vi "PicoScope4000SetupStreaming.vi"(0 "handle in":i16, 2 "enabled array":i16[](array[numeric]), 3 "Acquisition Settings":T2 {"Time Units" items=["Nanoseconds (ns)", "Microseconds (us)", "Milliseconds (ms)", "Seconds (s)"]; "Down-Sample Mode" items=["None", "Aggregate", "Decimate", "Average"]}, 4 "Buffer and Transfer Settings":T1 {"Down-Sample Mode" items=["None", "Aggregate", "Average"]; "Down Sample Ratio" step=1; "Samples" format="%_6p"}, 5 "error in":errorcluster, 10 "Pointers In":u64[][](array[numeric])) -> (11 "Pointer array":u64[][](array[numeric]), 14 "handle out":i16, 16 "Sample Interval":u32, 17 "sampleIntervalTimeUnits":u32, 19 "error out":errorcluster)   [LabVIEW 2009]
doc: "Set up the data buffers and calls RunStreaming to start the device streaming.\nData will be copied from the driver buffers into the corresponding application buffers using the wrapper dll."
uses:
  ps4000.dll
  ps4000Wrap.dll
  PicoScope4000Buffer and Transfer Settings.ctl
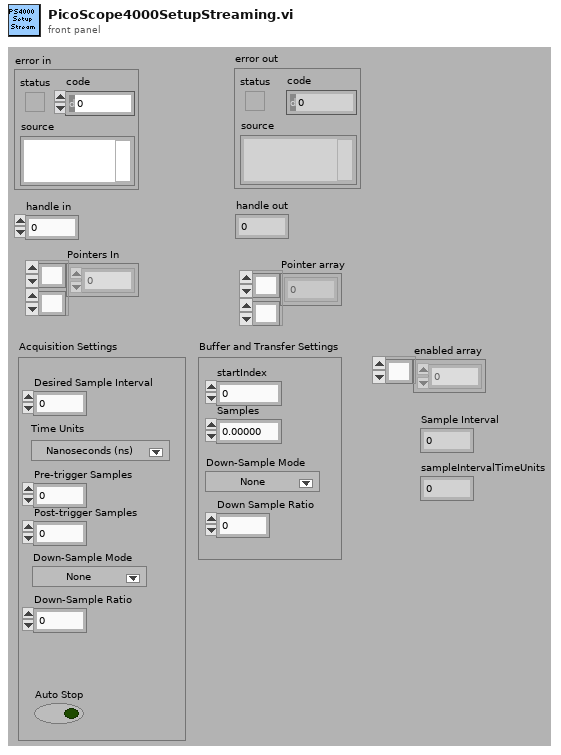
[diagram p1: front panel]
types:
  T1 = typedef "PicoScope4000Buffer and Transfer Settings.ctl" = cluster{"startIndex":u64, "Samples":u64, "Down Sample Ratio":u64, "Down-Sample Mode":u32}
  T2 = cluster{"Auto Stop":bool, "Desired Sample Interval":u32, "Pre-trigger Samples":u32, "Post-trigger Samples":u32, "Down-Sample Ratio":u32, "Down-Sample Mode":i32, "Time Units":u32}
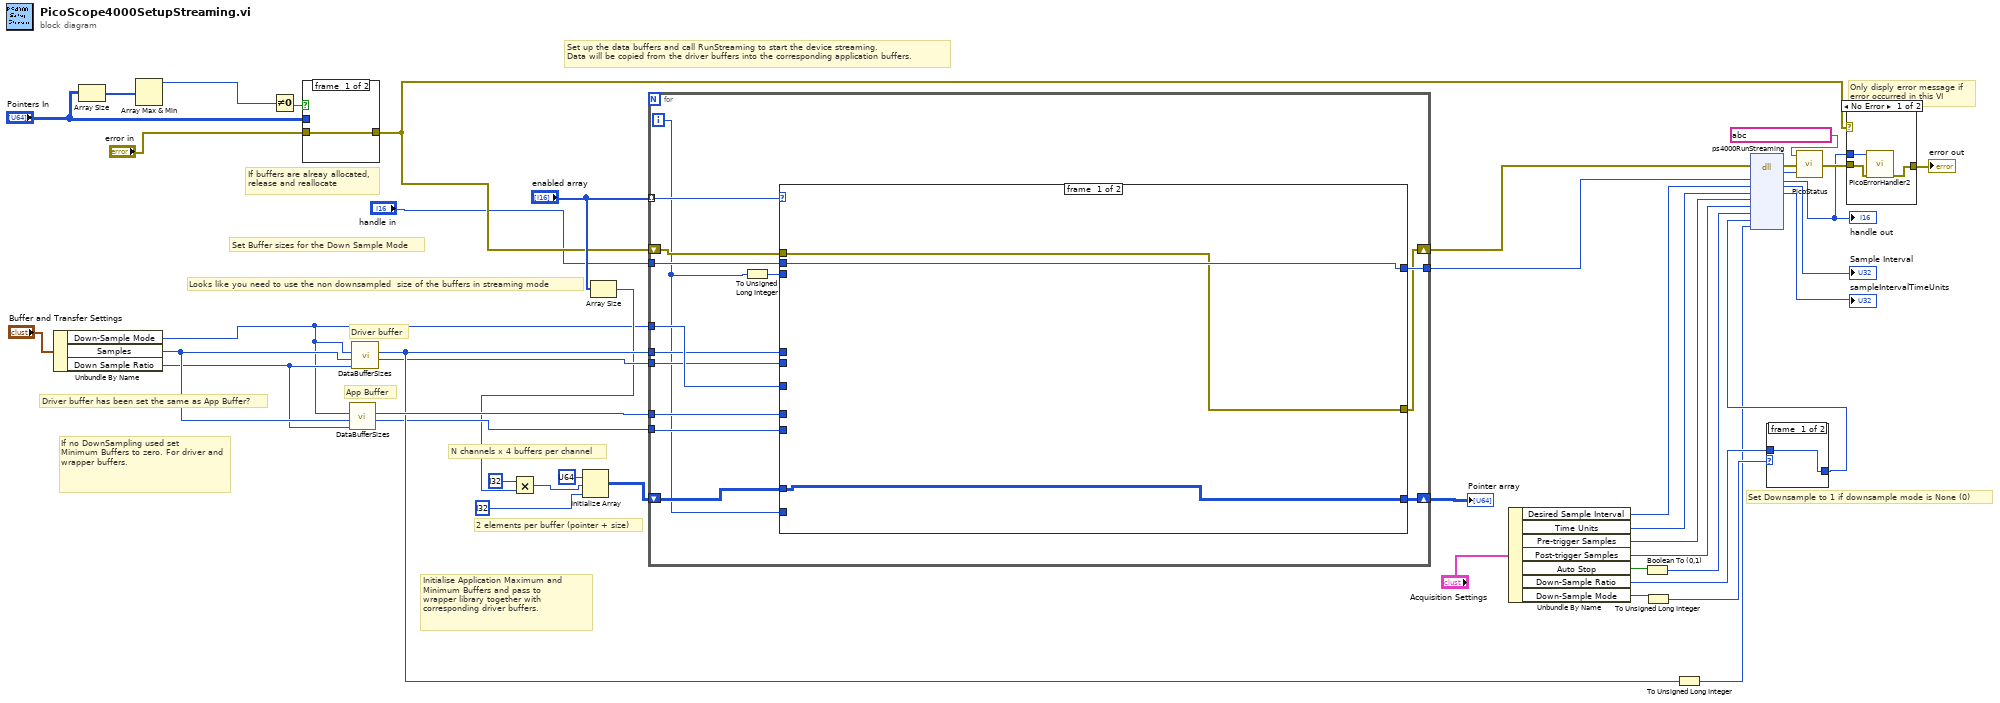
[diagram p0: block diagram]
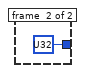
[diagram p2: hidden frame]
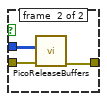
[diagram p3: hidden frame]
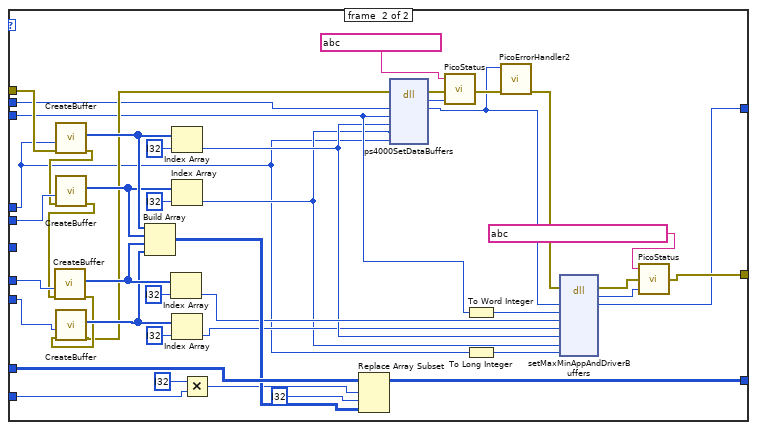
[diagram p4: hidden frame]
diagram:
  # "Set Downsample to 1 if downsample mode is None (0)"
  # "Looks like you need to use the non downsampled  size of the buffers in streaming mode"
  # "If buffers are alreay allocated,\nrelease and reallocate"
  # "2 elements per buffer (pointer + size)"
  # "N channels x 4 buffers per channel"
  # "App Buffer"
  # "Driver buffer"
  # "Driver buffer has been set the same as App Buffer?"
  # "Set Buffer sizes for the Down Sample Mode"
  # "If no DownSampling used set \nMinimum Buffers to zero. For driver and wrapper buffers."
  # "Initialise Application Maximum and\nMinimum Buffers and pass to \nwrapper library together with corresponding driver buffers."
  # "Only disply error message if\nerror occurred in this VI"
  # "Set up the data buffers and call RunStreaming to start the device streaming.\nData will be copied from the driver buffers into the corresponding application buffers."
  n1 = Unbundle By Name("Buffer and Transfer Settings") -> ("Down-Sample Mode"=w20:u32, "Samples"=w40:u64, "Down Sample Ratio"=w39:u64)
  n2 = Array Size(array="Pointers In") -> (size(s)=w22:i32[])
  n3 = Array Max & Min(array=w22) -> (max value=w21:i32)  [unwired: 3 out]
  n4 = Not Equal To 0?(x=w21) -> (x != 0?=w26:bool)
  n5 = case shown="True" w26 {
    tunnel: "Pointers In" -> [_ w47]
    tunnel: "error in" -> [w46 w48]
    tunnel: [w46 w49] -> w17
    frame #0 {
    }
    frame #1 {
      n6 = call "PicoReleaseBuffers.vi"("error in (no error)"=w48, "Pointer array"=w47) -> ("error out"=w49:errorcluster)  [unwired: 9 in]
    }
  }
  n7 = call "DataBufferSizes.vi"("Down Sample Ratio"=w39, "Number of Samples"=w40, "Down-Sample Mode"=w20) -> ("min Buffer Size"=w35:i32, "Max Buffer Size"=w38:i32)  [unwired: 7 in]
  n8 = call "DataBufferSizes.vi"("Down Sample Ratio"=w39, "Number of Samples"=w40, "Down-Sample Mode"=w20) -> ("min Buffer Size"=w36:i32, "Max Buffer Size"=w37:i32)  [unwired: 7 in]
  n9 = Array Size(array="enabled array") -> (size(s)=w29:i32)
  n10 = Multiply(x=i32 ?, y=w29) -> (x*y=w30:i32)
  n11 = Initialize Array(u64 ? ("element"), w30, i32 ? ("dimension size")) -> (w23:u64[][])
  n12 = for {
    tunnel: "enabled array" -> [w55] mode=indexing
    tunnel: "handle in" -> [w63]
    tunnel: w20 -> [w62]
    tunnel: w38 -> [w61]
    tunnel: w37 -> [w60]
    tunnel: w36 -> [w59]
    tunnel: w35 -> [w58]
    tunnel: [w56] -> w9
    shift-right: [w54] -> w1
    shift-left: w17 -> [w53]
    shift-right: [w57] -> w34
    shift-left: w23 -> [w52]
    i -> [w50]
    n13 = To Unsigned Long Integer(number=w50) -> (unsigned 32bit integer=w51:u32)
    n14 = case shown="1" w55 {
      tunnel: w63 -> [w65 w83]
      tunnel: w53 -> [w64 w88]
      tunnel: w51 -> [_ w81]
      tunnel: w61 -> [_ w89]
      tunnel: w60 -> [_ w68]
      tunnel: w59 -> [_ w104]
      tunnel: w58 -> [_ w103]
      tunnel: w62 -> [_ _]
      tunnel: w52 -> [w66 w98]
      tunnel: [w66 w97] -> w57
      tunnel: w50 -> [_ w95]
      tunnel: [w65 w74] -> w56
      tunnel: [w64 w91] -> w54
      frame #0 {
      }
      frame #1 {
        n15 = call "CreateBuffer.vi"("error in (no error)"=w88, "Buffer size"=w68) -> ("error out"=w87:errorcluster, "Pointer and BufferSize"=w102:u64[])  [unwired: 8 in]
        n16 = call "CreateBuffer.vi"("error in (no error)"=w87, "Buffer size"=w104) -> ("error out"=w86:errorcluster, "Pointer and BufferSize"=w101:u64[])  [unwired: 8 in]
        n17 = call "CreateBuffer.vi"("error in (no error)"=w86, "Buffer size"=w89) -> ("error out"=w85:errorcluster, "Pointer and BufferSize"=w100:u64[])  [unwired: 8 in]
        n18 = call "CreateBuffer.vi"("error in (no error)"=w85, "Buffer size"=w103) -> ("error out"=w84:errorcluster, "Pointer and BufferSize"=w99:u64[])  [unwired: 8 in]
        n19 = Build Array(w102, w101, w100, w99) -> (w94:u64[][])
        n20 = Index Array(array=w100, index=i32 ?) -> (element=w72:u64)
        n21 = Index Array(array=w102, index=i32 ?) -> (element=w71:u64)
        n22 = Index Array(array=w101, index=i32 ?) -> (element=w69:u64)
        n23 = Index Array(array=w99, index=i32 ?) -> (element=w70:u64)
        n24 = Multiply(x=i32 ?, y=w95) -> (x*y=w93:i32)
        n25 = Replace Array Subset(array=w98, new element=w94, index (row)=w93, index (col)=i32 ? ("disabled index (row)")) -> (w97:u64[][])
        n26 = dll-call lib="PS4000.dll" fn="ps4000SetDataBuffers" ("ps3000.dll:_ps3000_open_unit@0")(error in=w84, "handle"=w83, "channel"=w81, "bufferMax"=w71, "bufferMin"=w69, "bufferLth"=w68) -> (error out=w78:errorcluster, "PICO_STATUS"=w79:u32, "handle"=w73:i16)  [unwired: 6 in, 1 out]
        n27 = call "PicoStatus.vi"("PICO STATUS"=w79, "error in"=w78, "source"=string ?) -> ("error out"=w90:errorcluster)
        n28 = To Word Integer(number=w81) -> (16bit integer=w80:i16)
        n29 = To Long Integer(number=w68) -> (32bit integer=w82:i32)
        n30 = call "PicoErrorHandler2.vi"("error in (no error)"=w90, "handle In"=w73) -> ("error out"=w77:errorcluster)  [unwired: 9 in]
        n31 = dll-call lib="ps4000Wrap.dll" fn="setMaxMinAppAndDriverBuffers"(error in=w77, "handle"=w73, "channel"=w80, "appMaxBuffer"=w72, "appMinBuffer"=w70, "driverMaxBuffer"=w71, "driverMinBuffer"=w69, "bufferLength"=w82) -> (error out=w76:errorcluster, "PICO_STATUS"=w75:u32, "handle"=w74:i16)  [unwired: 8 in, 1 out]
        n32 = call "PicoStatus.vi"("PICO STATUS"=w75, "error in"=w76, "source"=string ?) -> ("error out"=w91:errorcluster)
      }
    }
  }
  "Pointer array" <- w34
  n33 = Unbundle By Name("Acquisition Settings") -> ("Desired Sample Interval"=w8:u32, "Time Units"=w7:u32, "Pre-trigger Samples"=w6:u32, "Post-trigger Samples"=w5:u32, "Auto Stop"=w43:bool, "Down-Sample Ratio"=w18:u32, "Down-Sample Mode"=w41:i32)
  n34 = Boolean To (0,1)(Boolean=w43) -> (0, 1=w4:i16)
  n35 = To Unsigned Long Integer(number=w41) -> (unsigned 32bit integer=w19:u32)
  n36 = To Unsigned Long Integer(number=w37) -> (unsigned 32bit integer=w2:u32)
  n37 = case shown="0" w19 {
    tunnel: [w110 u32 ? ("Down-Sample Ratio")] -> w3
    tunnel: w18 -> [w110 _]
    frame #0 {
    }
    frame #1 {
    }
  }
  n38 = dll-call lib="PS4000.dll" fn="ps4000RunStreaming" ("ps3000.dll:_ps3000_open_unit@0")(error in=w1, "handle"=w9, "sampleInterval"=w8, "sampleIntervalTimeUnits"=w7, "maxPreTriggerSamples"=w6, "maxPostTriggerSamples"=w5, "autoStop"=w4, "downSampleRatio"=w3, "overviewBufferSize"=w2) -> (error out=w14:errorcluster, "PICO_STATUS"=w13:u32, "handle"=w12:i16, "sampleInterval"=→"Sample Interval":u32, "sampleIntervalTimeUnits"=→"sampleIntervalTimeUnits":u32)  [unwired: 7 in, 1 out]
  "handle out" <- w12
  n39 = call "PicoStatus.vi"("PICO STATUS"=w13, "error in"=w14, "source"=string ?) -> ("error out"=w44:errorcluster)
  n40 = case shown="No Error" w17 {
    tunnel: [w113 w115] -> w45
    tunnel: w44 -> [w114 w115]
    tunnel: w12 -> [w112 _]
    frame #0 {
      n41 = call "PicoErrorHandler2.vi"("error in (no error)"=w114, "handle In"=w112) -> ("error out"=w113:errorcluster)  [unwired: 9 in]
    }
    frame #1 {
    }
  }
  "error out" <- w45
